vi "Get Default Headers.vi"(8 "error in (no error)":errorcluster, 11 "LabVIEWHTTPClient_NET in":refnum<class "HttpClient_NET.lvclass">) -> (0 "error out":errorcluster, 2 "DefaultRequest Headers":refnum<class "HttpHeaders_Request.lvclass">, 3 "LabVIEWHTTPClient_NET out":refnum<class "HttpClient_NET.lvclass">)   [LabVIEW 2018, in "HttpClient_NET.lvlib" / "HttpClient_NET.lvclass"]
doc: "DefaultRequestHeaders are run \"by ref\"\nand the lifetime is owned by the HTTP Client\nSo, it can be read here, and edited downstream with out need\nto \"rewrite\" it to the Client"
uses:
  HttpClient_NET.lvclass
  HttpHeaders_Request/HttpHeaders_Request.lvclass
  C:/Viviota/Projects/R&D/LabVIEW_HTTP_REST_NET/HTTPHeaders_NET/HttpHeaders_NET.lvclass
  HttpClient_NET.lvclass/HttpClient_NET.ctl
  System.Net.Http
  Accessors/Read NET_HttpClient.vi
  HTTPHeaders_NET/HttpHeaders_NET.lvclass
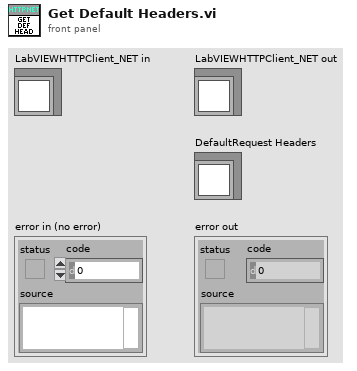
[diagram p1: front panel]
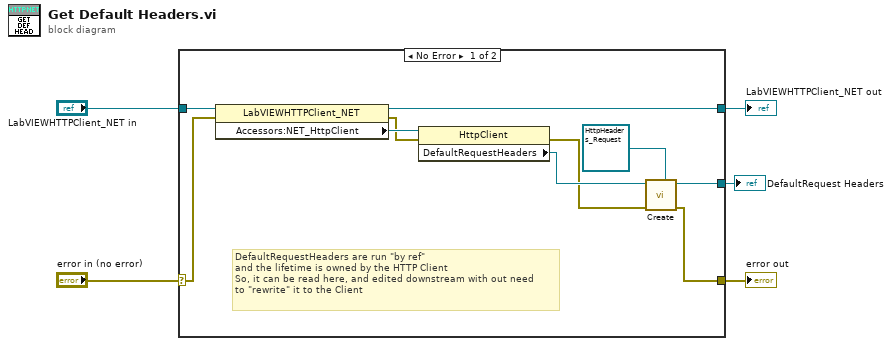
[diagram p0: block diagram]
diagram:
  n1 = case shown="No Error" "error in (no error)" {
    selector: "error in (no error)" -> [w9 w17]
    tunnel: [w6 w17] -> w4
    tunnel: [w14 w16] -> w2
    tunnel: "LabVIEWHTTPClient_NET in" -> [w15 w16]
    tunnel: [w10 _] -> w1
    frame No Error {
      # "DefaultRequestHeaders are run \"by ref\"\nand the lifetime is owned by the HTTP Client\nSo, it can be read here, and edited downstream with out need\nto \"rewrite\" it to the Client"
      n2 = property class="LabVIEWHTTPClient_NET"(reference=w15, error in=w9) -> (reference out=w14:refnum<class "HttpClient_NET.lvclass">, error out=w8:errorcluster, "Accessors:NET_HttpClient"=w12:refnum<k24>)
      n3 = property class="HttpClient"(reference=w12, error in=w8) -> (error out=w7:errorcluster, "DefaultRequestHeaders"=w11:refnum<k24>)  [unwired: 1 out]
      n4 = call "Create.vi"("HTTPHeaders_NET in"=refnum<class "HttpHeaders_Request.lvclass"> refnum ("LabVIEWHTTPClient_NET.lvlib:HttpHeaders_Request.lvclass"), "error in (no error)"=w7, "NET_HttpHeaders"=w11) -> ("error out"=w6:errorcluster, "HTTPHeaders_NET out"=w10:refnum<class "HttpHeaders_Request.lvclass">)  [unwired: 7 in]
    }
    frame Error {
    }
  }
  "error out" <- w4
  "LabVIEWHTTPClient_NET out" <- w2
  "DefaultRequest Headers" <- w1
